vi "REV Degrees to Rotations.vi"() -> ()   [LabVIEW 2020]
panel:
  out "rotations":dbl
  in  "degrees":dbl
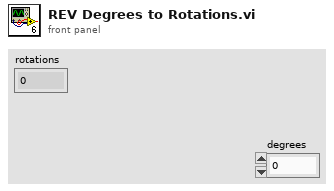
[diagram p1: front panel]
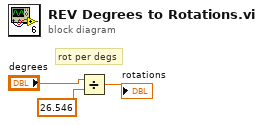
[diagram p0: block diagram]
diagram:
  # "rot per degs"
  n1 = Divide(x="degrees", y=26.546) -> (x/y=→"rotations":dbl)
